vi "Edit Legend.vi"(8 "Error In":errorcluster, 9 "Maximum String Length":i32=12, 10 "channel name(s)":string[](array[string]), 11 "Graph Ref In":refnum<vi>) -> (0 "Error Out":errorcluster, 3 "Graph Ref Out":refnum<vi>)   [LabVIEW 2019, in "Graph Tools.lvlib"]
doc: "Update Graph Legend and limit number of characters if a channel name is to long."
uses:
  Graph Tools.lvlib
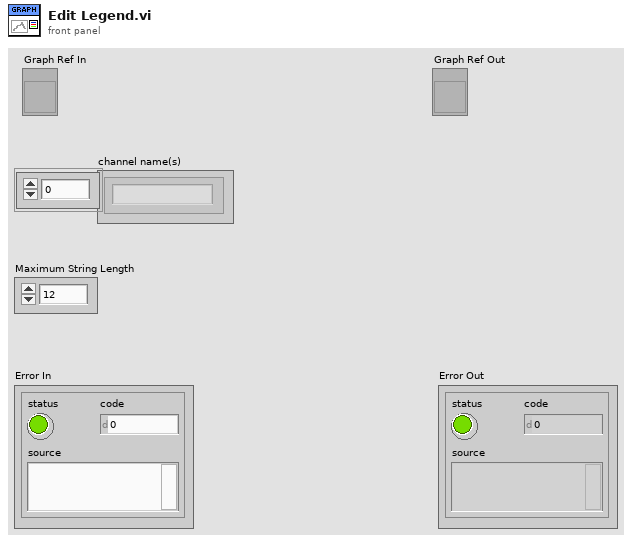
[diagram p1: front panel]
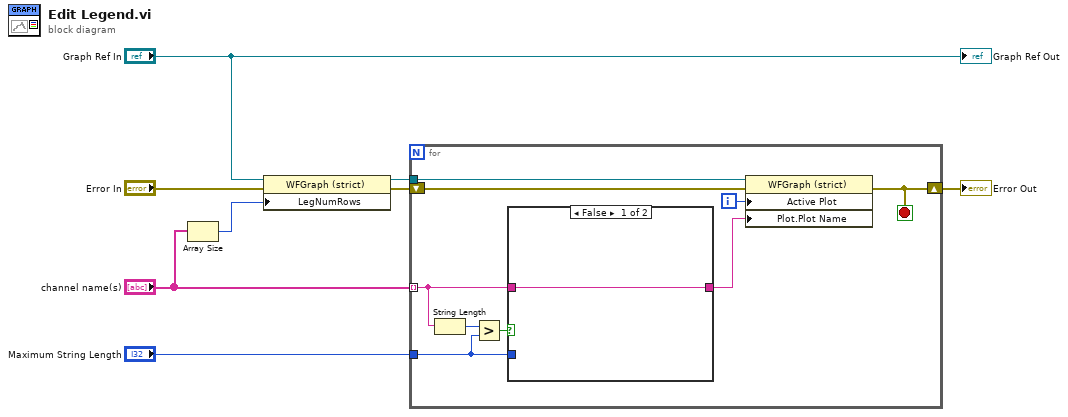
[diagram p0: block diagram]
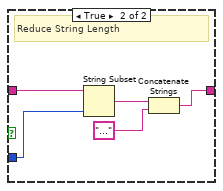
[diagram p2: hidden frame]
diagram:
  n1 = Array Size(array="channel name(s)") -> (size(s)=w6:i32)
  n2 = property on="Property Node" class="WFGraph (strict)"(reference="Graph Ref In", error in="Error In", "LegNumRows"=w6) -> (reference out=w7:refnum<vi>, error out=w8:errorcluster)
  n3 = for {
    tunnel: "channel name(s)" -> [w12] mode=indexing
    shift-right: [w15] -> w3
    shift-left: w8 -> [w16]
    tunnel: w7 -> [w14]
    tunnel: "Maximum String Length" -> [w10]
    i -> [w17]
    stop <- w15 stop-if-true
    n4 = String Length(string=w12) -> (length=w9:i32)
    n5 = Greater?(x=w9, y=w10) -> (0:w11:bool)
    n6 = case shown="False" w11 {
      tunnel: [w18 w21] -> w13
      tunnel: w12 -> [w18 w22]
      tunnel: w10 -> [_ w19]
      frame False {
      }
      frame True {
        # "Reduce String Length"
        n7 = String Subset(string=w22, length (rest)=w19) -> (substring=w23:string)  [unwired: 1 in]
        n8 = Concatenate Strings(w23, "..." ("string")) -> (w21:string)
      }
    }
    n9 = property on="Property Node" class="WFGraph (strict)"(reference=w14, error in=w16, "Active Plot"=w17, "Plot.Plot Name"=w13) -> (error out=w15:errorcluster)  [unwired: 1 out]
  }
  "Error Out" <- w3
  "Graph Ref Out" <- "Graph Ref In"
